vi "Player Info.vi"(8 "Victory Speech":string="Wow, I won??", 9 "Name":string="Explorer", 11 "Explorer in":refnum<class "Explorer.lvclass">) -> (3 "Explorer out":refnum<class "Explorer.lvclass">)   [LabVIEW 2015, in "Explorer.lvclass"]
uses:
  Explorer.lvclass
  Square/Square.lvclass
panel:
  # "Set default values for these two string controls"
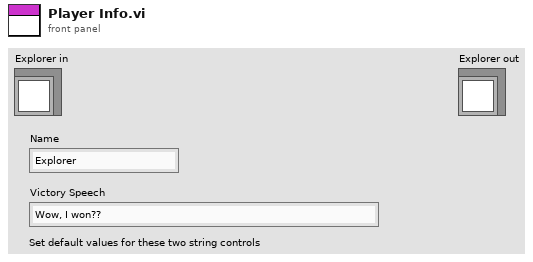
[diagram p1: front panel]
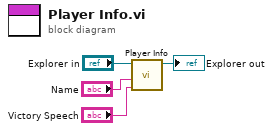
[diagram p0: block diagram]
diagram:
  n1 = call-parent "Player Info.vi"("Victory Speech"="Victory Speech", "Name"="Name", "Square in"="Explorer in") -> ("Square out"=→"Explorer out":refnum<class "Explorer.lvclass">)  [unwired: 8 in]
